vi "Siglent SDS 1000 2000 Series Acquire Waveform In Loop.vi"() -> ()   [LabVIEW 2021]
doc: "This example shows how to use autosetup and acquire a waveform on a single channel for acquiring waveforms in a loop until stopped by user."
uses:
  <instrlib>/Siglent SDS 1000 2000 Series/Public/Data/Read Waveform (Single).vi
  <instrlib>/Siglent SDS 1000 2000 Series/Siglent SDS 1000 2000 Series.lvlib
panel:
  in  "Reset (True)":bool=TRUE
  in  "Perform Auto Setup":bool
  in  "Timeout (10000 ms)":u32=10000
  in  "Source (1: Channel 1)":u16(ring)=1 items=["Channel 1"=1, "Channel 2"=2, "Channel 3"=3, "Channel 4"=4]
  in  "STOP":bool
  out "Waveform Data":waveform(dbl)(graph)
  in  "VISA resource name":refnum<visa-resource-name>
  # "(c) 2015 SIGLENT TECHNOLOGIES CO., LTD.   ALL RIGHTS RESERVED."
  # "Directions:\n\n1. Setup the scope to be able to successfully single trigger on a signal applied to the channel selected in the \"Source\" control,  or set Perform Auto Setup? to True to perform an autosetup. \n\n2. On this front panel, enter the VISA Resource name for your scope. (e.g. VICP::123.45.67.8 for TCP/IP, GPIB::5::INSTR for GPIB). Modify the timeout if necessary.\n\n3. For an initial test, set the Reset? and Perform Auto Setup? controls to True, and then run the VI to find the signal.  Leave both set to False for subsequent runs."
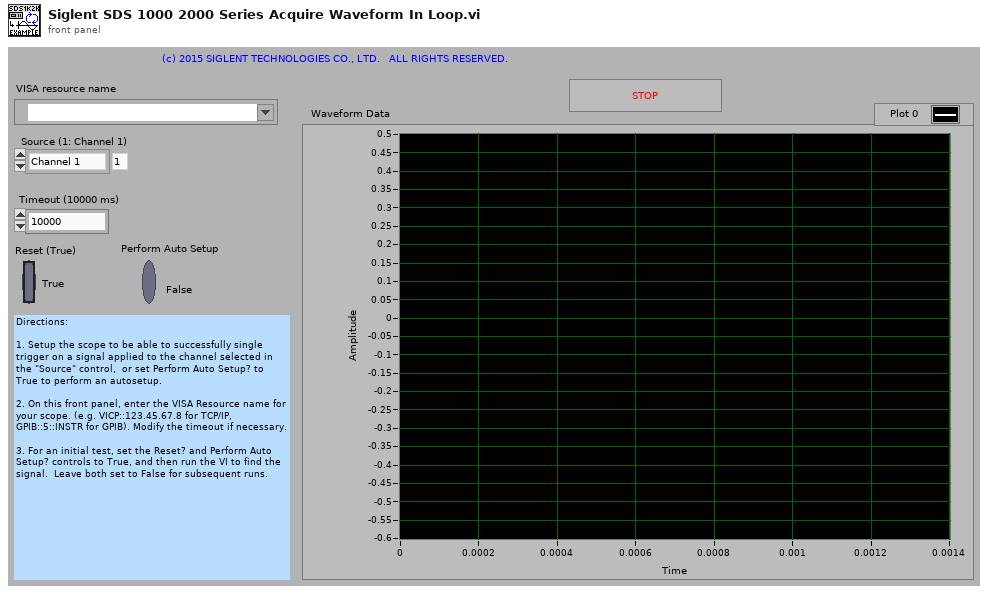
[diagram p1: front panel]
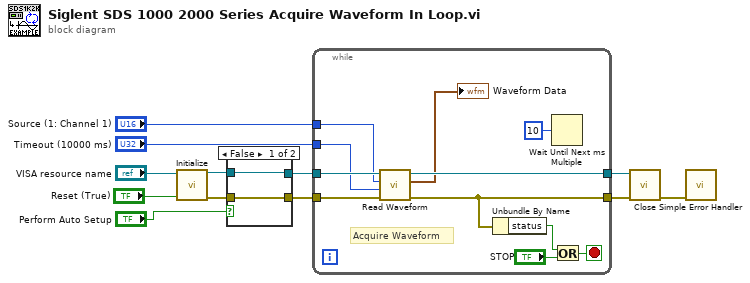
[diagram p0: block diagram]
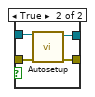
[diagram p2: hidden frame]
diagram:
  n1 = call <instrlib>:"Initialize.vi"("Reset (True)"="Reset (True)", "VISA resource name"="VISA resource name") -> ("error out"=w8:errorcluster, "VISA resource name out"=w7:refnum<visa-resource-name>)  [unwired: 8 in]
  n2 = case shown="False" "Perform Auto Setup" {
    tunnel: w8 -> [w13 w18]
    tunnel: w7 -> [w14 w17]
    tunnel: [w14 w16] -> w6
    tunnel: [w13 w15] -> w5
    frame False {
    }
    frame True {
      n3 = call <instrlib>:"Autosetup.vi"("error in (no error)"=w18, "VISA resource name"=w17) -> ("error out"=w15:errorcluster, "VISA resource name out"=w16:refnum<visa-resource-name>)  [unwired: 8 in]
    }
  }
  n4 = while {
    tunnel: w6 -> [w29]
    tunnel: w5 -> [w28]
    tunnel: [w27] -> w11
    tunnel: [w24] -> w10
    tunnel: "Source (1: Channel 1)" -> [w21]
    tunnel: "Timeout (10000 ms)" -> [w20]
    stop <- w25 stop-if-true
    # "Acquire Waveform"
    n5 = call-poly <instrlib>:"Read Waveform.vi"("error in (no error)"=w28, "Timeout (10000 ms)"=w20, "Source (1: Channel 1)"=w21, "VISA resource name"=w29) -> ("error out"=w24:errorcluster, "Waveform Data"=→"Waveform Data":waveform(dbl), "VISA resource name out"=w27:refnum<visa-resource-name>)  [unwired: 5 in]
    n6 = Unbundle By Name(w24) -> ("status"=w23:bool)
    n7 = Wait Until Next ms Multiple(millisecond multiple=u32 10) -> ()  [unwired: 1 out]
    n8 = Or(x=w23, y="STOP") -> (x .or. y?=w25:bool)
  }
  n9 = call <instrlib>:"Close.vi"("error in (no error)"=w10, "VISA resource name"=w11) -> ("error out"=w12:errorcluster)  [unwired: 9 in]
  n10 = call <vilib>:"Simple Error Handler.vi"("error in (no error)"=w12) -> ()  [unwired: 4 in, 5 out]
